vi "Sig2MS getSignalInfo.vi"(8 "error in (no error)":errorcluster, 11 "Sig2MS in":refnum<class "Sig2MS.lvclass">) -> (0 "error out":errorcluster, 2 "pySigFormat":T1, 3 "Sig2MS out":refnum<class "Sig2MS.lvclass">)   [LabVIEW 2018, in "Sig2MS.lvclass"]
uses:
  Sig2MS.lvclass
  Sig2MS.lvclass/Sig2MS.ctl
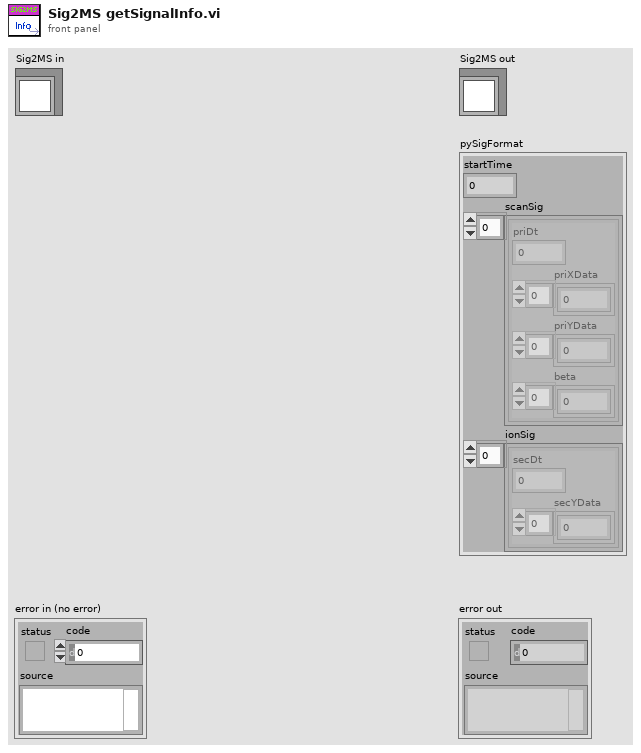
[diagram p1: front panel]
types:
  T1 = cluster{"startTime":dbl, "scanSig":cluster{"priDt":dbl, "priXData":dbl[], "priYData":sgl[], "beta":dbl[]}[], "ionSig":cluster{"secDt":dbl, "secYData":sgl[]}[]}
  T2 = cluster{"priDt":dbl, "priXData":dbl[], "priYData":sgl[], "beta":dbl[]}[]
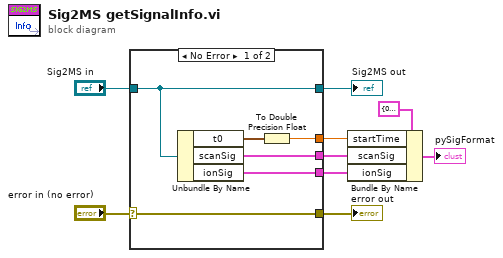
[diagram p0: block diagram]
diagram:
  n1 = case shown="No Error" "error in (no error)" {
    selector: "error in (no error)" -> [w14 w17]
    tunnel: [w14 w17] -> w8
    tunnel: [w15 w16] -> w6
    tunnel: "Sig2MS in" -> [w15 w16]
    tunnel: [w12 _] -> w4
    tunnel: [w11 _] -> w3
    tunnel: [w10 _] -> w2
    frame No Error {
      n2 = Unbundle By Name(w15) -> ("t0"=w13:timestamp, "scanSig"=w11:T2, "ionSig"=w10:cluster{"secDt":dbl, "secYData":sgl[]}[])
      n3 = To Double Precision Float(number=w13) -> (double precision float=w12:dbl)
    }
    frame Error {
    }
  }
  "error out" <- w8
  "Sig2MS out" <- w6
  n4 = Bundle By Name(cluster=T1 {"startTime"=0.0, "scanSig"=[], "ionSig"=[]} ("sigData"), "startTime"=w4, "scanSig"=w3, "ionSig"=w2) -> (→"pySigFormat":T1)
